vi "Plugin Options Dialog.vi"(8 "error in (no error)":errorcluster, 11 "Application in":refnum<data-value>) -> (0 "error out":errorcluster, 3 "Application out":refnum<data-value>)   [LabVIEW 2015, in "Application.lvclass"]
uses:
  Application.lvclass
  Plugin Options UI State.ctl
  Plugin.lvclass
panel:
  in  "Plugin":i32(listbox)
  in  "Cancel Btn":bool
  in  "Save Btn":bool
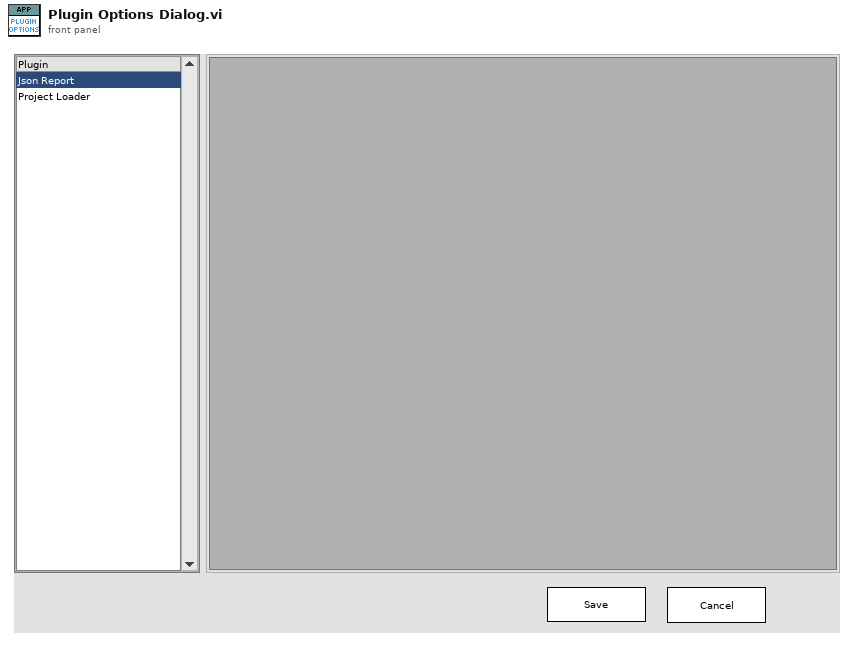
[diagram p1: front panel]
types:
  T1 = cluster{"Plugin Options":refnum<vi>, "Config VI":refnum<vi>, "Plugin":i32, "Save":bool}
  T2 = typedef "Application.lvclass/Plugin Options UI State.ctl" = enum16{"UI_LOOP", "INIT", "EXIT", "PLUGIN_CHANGE"}
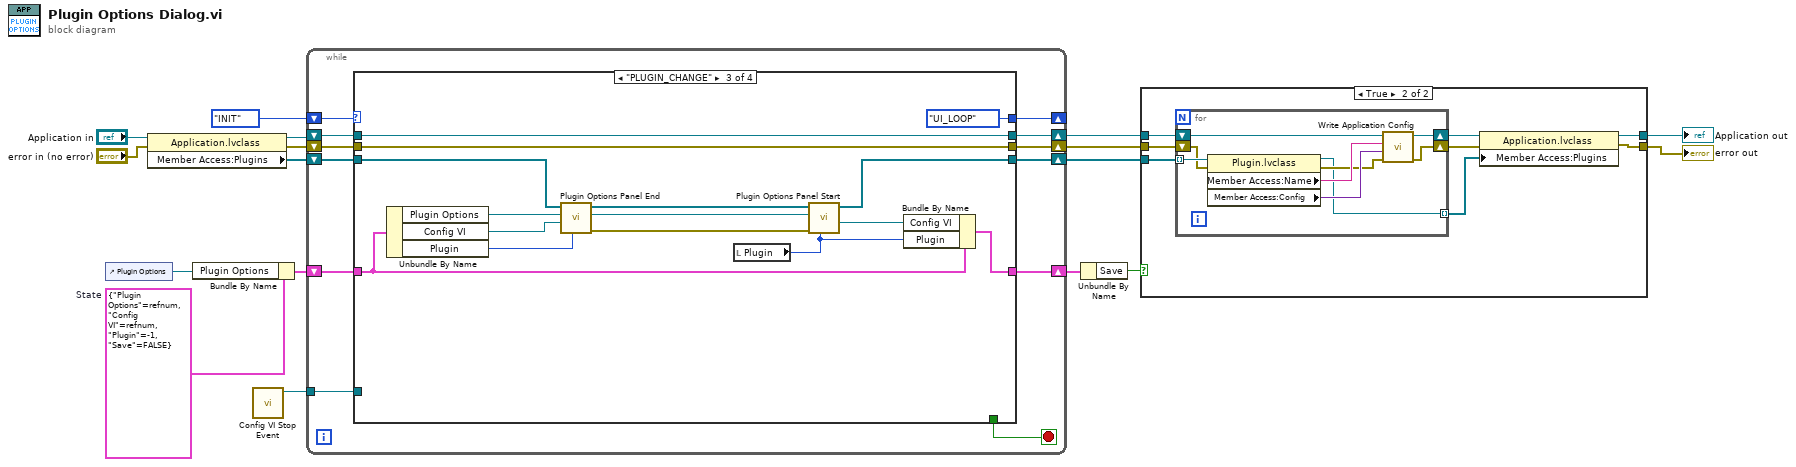
[diagram p0: block diagram]
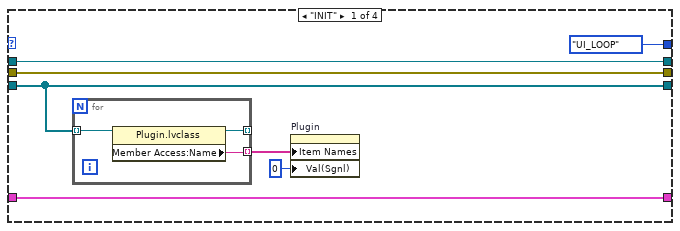
[diagram p2: hidden frame]
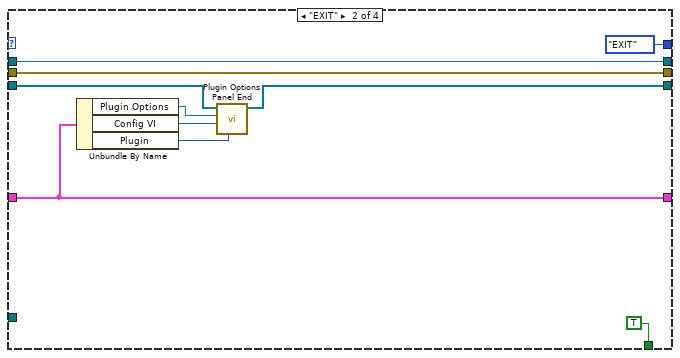
[diagram p3: hidden frame]
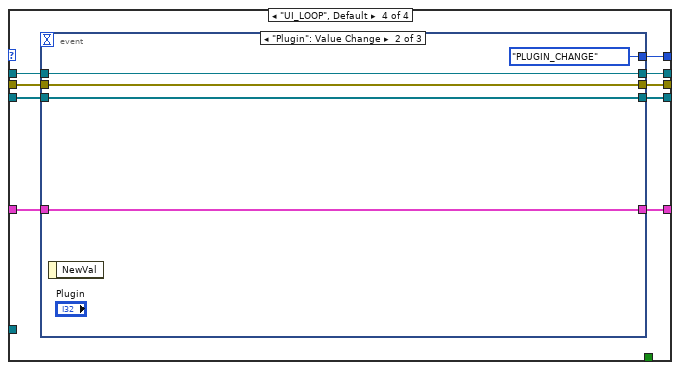
[diagram p4: hidden frame]
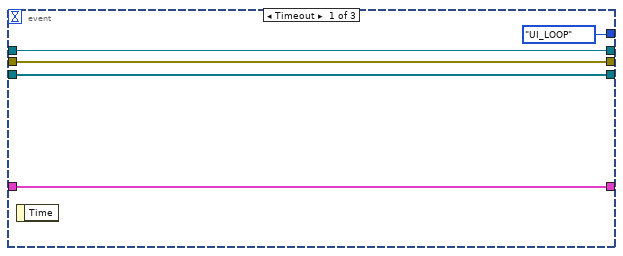
[diagram p5: hidden frame]
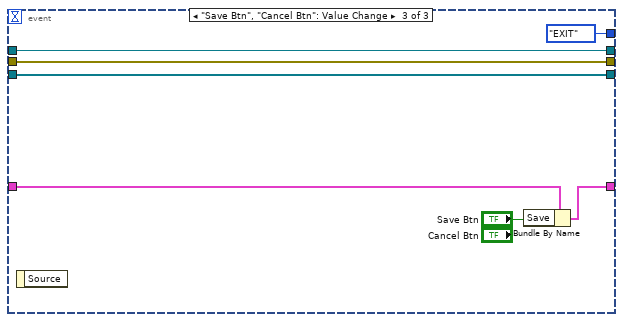
[diagram p6: hidden frame]
diagram:
  w5 = T1 {"Plugin Options"=refnum, "Config VI"=refnum, "Plugin"=-1, "Save"=FALSE}  # State
  n1 = control-ref of="Plugin Options"() -> (w4:refnum<vi>)
  n2 = property class="Application.lvclass"(reference="Application in", error in="error in (no error)") -> (reference out=w15:refnum<data-value>, error out=w12:errorcluster, "Member Access:Plugins"=w14:refnum<class "Plugin.lvclass">[])
  n3 = Bundle By Name(cluster=w5, "Plugin Options"=w4) -> (w3:T1)
  n4 = call "Config VI Stop Event.vi"() -> ("VI Stop event"=w11:refnum<user-event>)  [unwired: 11 in]
  n5 = while {
    shift-right: [w24] -> _
    shift-left: Plugin_Options_UI_State."INIT" -> [w29]
    shift-right: [w27] -> w10
    shift-left: w15 -> [w28]
    shift-right: [w25] -> w8
    shift-left: w14 -> [w26]
    shift-right: [w21] -> w9
    shift-left: w12 -> [w22]
    tunnel: w11 -> [w20]
    shift-right: [w19] -> w2
    shift-left: w3 -> [w18]
    stop <- w23 stop-if-true
    n6 = case shown="\"PLUGIN_CHANGE\"" w29 {
      tunnel: w28 -> [w36 w49 w63 w72]
      tunnel: [w36 w49 w63 w71] -> w27
      tunnel: w26 -> [w34 w41 w54 w70]
      tunnel: [w34 w40 w52 w69] -> w25
      tunnel: [Plugin_Options_UI_State."UI_LOOP" Plugin_Options_UI_State."EXIT" Plugin_Options_UI_State."UI_LOOP" w73] -> w24
      tunnel: [_ TRUE _ _] -> w23
      tunnel: w22 -> [w32 w46 w62 w68]
      tunnel: [w32 w46 w62 w67] -> w21
      tunnel: w20 -> [_ _ _ _]
      tunnel: [w30 w43 w55 w65] -> w19
      tunnel: w18 -> [w30 w43 w57 w66]
      frame "INIT" {
        n7 = for {
          tunnel: w34 -> [w39] mode=indexing
          tunnel: [w38] -> w35 mode=indexing
          tunnel: [w37] -> _ mode=indexing
          n8 = property class="Plugin.lvclass"(reference=w39) -> (reference out=w37:refnum<class "Plugin.lvclass">, "Member Access:Name"=w38:string)  [unwired: 1 in, 1 out]
        }
        n9 = property on="Plugin" class="LstBox (strict)"("Item Names"=w35, "Val(Sgnl)"=0 ("Value (Signaling)")) -> ()  [unwired: 2 in, 2 out]
      }
      frame "EXIT" {
        n10 = Unbundle By Name(w43) -> ("Plugin Options"=w45:refnum<vi>, "Config VI"=w44:refnum<vi>, "Plugin"=w42:i32)
        n11 = call "Plugin Options Panel End.vi"("Index in"=w42, "Config VI Refnum in"=w44, "Container in"=w45, "Plugins in"=w41) -> ("Plugins out"=w40:refnum<class "Plugin.lvclass">[])  [unwired: 5 in, 2 out]
      }
      frame "PLUGIN_CHANGE" {
        n12 = Unbundle By Name(w57) -> ("Plugin Options"=w59:refnum<vi>, "Config VI"=w58:refnum<vi>, "Plugin"=w50:i32)
        n13 = call "Plugin Options Panel End.vi"("Index in"=w50, "Config VI Refnum in"=w58, "Container in"=w59, "Plugins in"=w54) -> ("error out"=w61:errorcluster, "Container out"=w60:refnum<vi>, "Plugins out"=w53:refnum<class "Plugin.lvclass">[])  [unwired: 5 in]
        n14 = local read "Plugin"() -> (w51:i32)
        n15 = call "Plugin Options Panel Start.vi"("Index in"=w51, "error in (no error)"=w61, "Container"=w60, "Plugins in"=w53) -> ("Config VI Refnum out"=w56:refnum<vi>, "Plugins out"=w52:refnum<class "Plugin.lvclass">[])  [unwired: 5 in, 1 out]
        n16 = Bundle By Name(cluster=w57, "Config VI"=w56, "Plugin"=w51) -> (w55:T1)
      }
      frame "UI_LOOP", Default {
        n17 = event shown="[1] \"Plugin\": Value Change" {
          selector: _ -> [_ _ _]
          dyn-events: _ -> [_ _ _]
          timeout: _ -> [_ _ _]
          tunnel: [Plugin_Options_UI_State."UI_LOOP" Plugin_Options_UI_State."PLUGIN_CHANGE" Plugin_Options_UI_State."EXIT"] -> w73
          tunnel: w72 -> [w77 w82 w89]
          tunnel: [w77 w82 w89] -> w71
          tunnel: w70 -> [w78 w83 w88]
          tunnel: [w78 w83 w88] -> w69
          tunnel: w68 -> [w75 w80 w87]
          tunnel: [w75 w80 w87] -> w67
          tunnel: w66 -> [w74 w79 w86]
          tunnel: [w74 w79 w85] -> w65
          event Timeout {
            n18 = event-data() -> ()  [unwired: 1 in, 1 out]
          }
          event "Plugin": Value Change {
            n19 = event-data() -> ()  [unwired: 1 in, 1 out]
          }
          event "Save Btn", "Cancel Btn": Value Change {
            n20 = event-data() -> ()  [unwired: 1 in, 1 out]
            n21 = Bundle By Name(cluster=w86, "Save"="Save Btn") -> (w85:T1)
          }
        }
      }
    }
  }
  n22 = Unbundle By Name(w2) -> ("Save"=w1:bool)
  n23 = case shown="True" w1 {
    tunnel: w10 -> [w92 w98]
    tunnel: w9 -> [w91 w97]
    tunnel: w8 -> [_ w96]
    tunnel: [w92 w100] -> w7
    tunnel: [w91 w99] -> w6
    frame False {
    }
    frame True {
      n24 = for {
        tunnel: w96 -> [w108] mode=indexing
        shift-right: [w103] -> w95
        shift-left: w98 -> [w109]
        shift-right: [w102] -> w94
        shift-left: w97 -> [w107]
        tunnel: [w101] -> w93 mode=indexing
        n25 = property class="Plugin.lvclass"(reference=w108, error in=w107) -> (reference out=w101:refnum<class "Plugin.lvclass">, error out=w104:errorcluster, "Member Access:Name"=w106:string, "Member Access:Config"=w105:variant)
        n26 = call "Write Application Config.vi"("error in (no error)"=w104, "Config Type In"=w105, "Section"=w106, "Application in"=w109) -> ("error out"=w102:errorcluster, "Application out"=w103:refnum<data-value>)  [unwired: 6 in]
      }
      n27 = property class="Application.lvclass"(reference=w95, error in=w94, "Member Access:Plugins"=w93) -> (reference out=w100:refnum<data-value>, error out=w99:errorcluster)
    }
  }
  "error out" <- w6
  "Application out" <- w7
